vi "TagBus_Write_DELETEME.vi"(9 "Value Array":dbl[](array[numeric]), 10 "Tag Key Array":string[](array[string])=["Load_kW", "EnergyStorage_kW", "Grid_kW"], 11 "TagBus.lvclass":refnum<class "TagBus.lvclass">) -> (3 "TagBus.lvclass out":refnum<class "TagBus.lvclass">)   [LabVIEW 2015]
uses:
  TagBus.lvclass
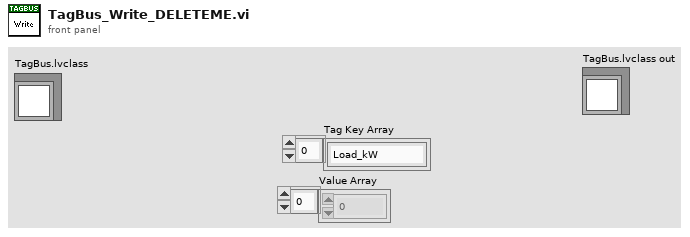
[diagram p1: front panel]
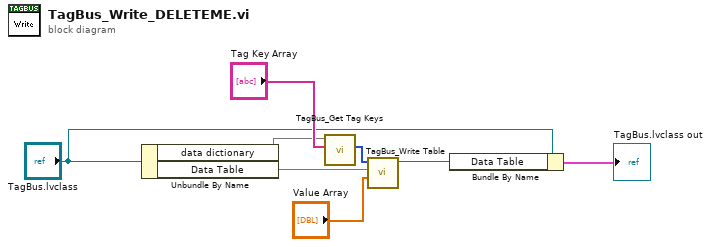
[diagram p0: block diagram]
diagram:
  n1 = Unbundle By Name("TagBus.lvclass") -> ("data dictionary"=w5, "Data Table"=w6)
  n2 = call "TagBus_Get Tag Keys.vi"("Tag Keys"="Tag Key Array", "TagBus"=w5) -> ("Index Array"=w7:i32[])  [unwired: 8 in, 1 out]
  n3 = call "TagBus_Write Table.vi"("Value Array"="Value Array", "Index Array"=w6, "TagBus in"=w7) -> ("TagBus out"=w4:refnum<class "TagBus.lvclass">)  [unwired: 8 in]
  n4 = Bundle By Name(cluster="TagBus.lvclass", "Data Table"=w4) -> (→"TagBus.lvclass out":cluster{})
